vi "Main Loop.vi"(8 "error in (no error)":errorcluster, 10 "Chart Notifier":refnum<notifier>, 11 "Message Queues":T1) -> (0 "error out":errorcluster)   [LabVIEW 2018, in "Sonicator Module.lvlib" / "Sonicator Module Engine.lvlib"]
uses:
  Sonicator Module Engine.lvlib
  Sonicator Message Queues.ctl
  support/Message Queue/Message Cluster.ctl
  Feed Module/Controls/Sonicator Module Display.ctl
  Feed Module/Controls/Sonicator Module State Cluster.ctl
  Pump Module Folder/Measure Instrument/State Enum.ctl
  Feed Module/Controls/Sonicator Module Config Cluster.ctl
  <vilib>/Utility/miscctls.llb/LVPoint32TypeDef.ctl
  Feed Module/Controls/Sonicator Module Settings Cluster.ctl
  Sonic Systems P100/Sonic Systems P100 Settings.ctl
  <vilib>/Platform/TimedLoop/XDataNode/timing_clust.ctl
  <vilib>/Platform/TimedLoop/XDataNode/nitl_modes.ctl
  <vilib>/Platform/TimedLoop/XDataNode/wakeup.ctl
  Tag VIs/Tag FGV Operation Enum.ctl
  support/Message Queue/Enqueue Message (Single).vi
  <vilib>/Platform/TimedLoop/XDataNode/XDataNode.xnode
  support/Message Queue/Message Queue.lvlib
  <vilib>/Platform/TimedLoop/XDataNode/XDNodeRunTimeDep.lvlib
  Sonicator Module.lvlib
  Shared Variables/Dynamic Shared Variables.lvlib
  support/Support Library.lvlib
  Sonic Systems P100/Sonic Systems P100.lvlib
  Pump Module Folder/Measure Instrument/Pump Module Engine.lvlib
panel:
  out "Period (s) 2":dbl format="%_4g"
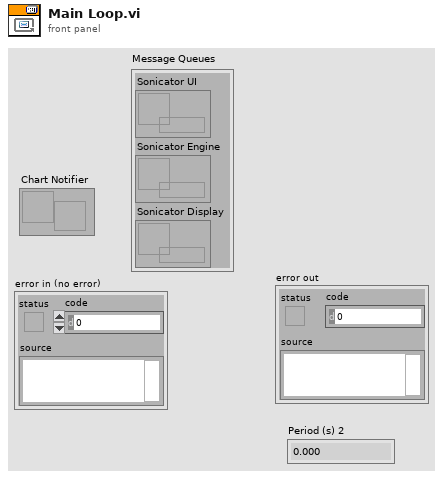
[diagram p1: front panel]
types:
  T1 = typedef "Sonicator Module.lvlib/Sonicator Message Queues.ctl" = cluster{"Sonicator UI":refnum<queue>, "Sonicator Engine":refnum<queue>, "Sonicator Display":refnum<queue>}
  T2 = typedef "XDNodeRunTimeDep.lvlib/timing_clust.ctl" = cluster{"Expected End [f-1]":u64, "Actual End [f-1]":u64, "Finished Late? [f-1]":bool, "Expected End [i-1]":u64, "Actual End [i-1]":u64, "Finished Late? [i-1]":bool, "Expected Start [i]":u64, "Actual Start [i]":u64, "Expected Start [f]":u64, "Actual Start [f]":u64, "Source Name":string, "Structure Name":string, "Period":i64, "Deadline":i64, "Offset":i64, "Start":i64, "Priority":i32, "Timeout":i32, "Mode":T3, "Wakeup Reason":T4, "Error":errorcluster, "Source Type":string, "Secondary Source Type":string, "Global End Time":u64, "Global Start Time":u64, "Frame Duration":u64, "Iteration Duration":u64, "Assigned CPU":i32, "I/O Scan Engine Mode":u32}
  T3 = typedef "XDNodeRunTimeDep.lvlib/nitl_modes.ctl" = enum32{"No Change", "Process missed periods, maintain original phase", "Discard missed periods, maintain original phase", "Process missed periods, ignore original phase", "Discard missed periods, ignore original phase"}
  T4 = typedef "XDNodeRunTimeDep.lvlib/wakeup.ctl" = enum32{"Normal", "Aborted", "Asynchronous wakeup", "Timing source error", "Timed loop error", "Timeout"}
  T5 = cluster{"enable? (F)":bool, "name":string, "alarm on":bool, "priority":u32, "ack type":enum16{"Auto", "User", "None", "Each Occurrence"}, "area":string, "description":string, "log? (T)":bool}
  T6 = typedef "Tag FGV Operation Enum.ctl" = enum16{"Init", "Set Notification Queue", "Create Tag", "Commit", "Write Tag (Numeric)", "Write Tag (Boolean)", "Read All Tags", "Read One Tag", "Delete Tag Category", "Set Alarm Parameters (Numeric)", "Set Alarm Parameters (Boolean)", "Enable All Alarms", "Disable All Alarms", "Delete All Tags", "Read Alarms", "Ack Alarm", "Read Alarm Parameters (Numeric)", "Read Alarm Parameters (Boolean)"}
  T7 = enum32{"u32BitField", "bool", "double", "string", "int8", "uint8", "int16", "uint16", "int32", "uint32", "int64", "uint64", "single", "double waveform", "int16 waveform", "array of boolean", "array of int8", "array of uint8", "array of int16", "array of uint16", "array of int32", "array of uint32", "array of int64", "array of uint64", "array of single", "array of double", "array of double waveform", "array of int16 waveform", "array of string", "variant", "timestamp", "fixed point", "custom"}
  T8 = typedef "Pump Module.lvlib/Pump Module Engine.lvlib/State Enum.ctl" = enum16{"Measuring", "Idle", "Paused"}
  T9 = enum16{"Off", "On", "Not Initialized", "Over Cutoff"}
  T10 = typedef "Sonicator Module.lvlib/Sonicator Module Config Cluster.ctl" = cluster{"GUID":string, "Drop Coords":T11, "Process Name":string, "User name":string, "Queue Name":string, "Settings":T12, "Load Count":i32}
  T11 = typedef "LVPoint32TypeDef.ctl" = cluster{"Horizontal":i32, "Vertical":i32}
  T12 = typedef "Sonicator Module.lvlib/Sonicator Module Settings Cluster.ctl" = cluster{"Cycle Period":dbl, "Sonicator Type":string, "SS P100 Settings":T13, "Setpoint (µm)":dbl, "Cutoff (W)":dbl}
  T13 = typedef "Sonic Systems P100.lvlib/Sonic Systems P100 Settings.ctl" = cluster{"VISA resource name":refnum<visa-resource-name>, "Simulated?":bool}
  T14 = typedef "Sonicator Module.lvlib/Sonicator Module State Cluster.ctl" = cluster{"State":T8, "Start Time":timestamp, "Current Time":timestamp, "Sonicator Module Config":T10, "Output Error":bool, "Log Started":bool, "First Iteration":bool, "Data":cluster{"Sonicator Amp Value":dbl, "Sonicator Power Value":dbl}, "Sonicator On?":enum16{"Off", "On", "Not Initialized", "Over Cutoff"}}
  T15 = typedef "Sonicator Module.lvlib/Sonicator Module Display.ctl" = cluster{"Sonicator On?":enum16{"Off", "On", "Not Initialized", "Over Cutoff"}, "Sonicator Amp Value":dbl, "Sonicator Power Value":dbl, "Cycle Period":dbl}
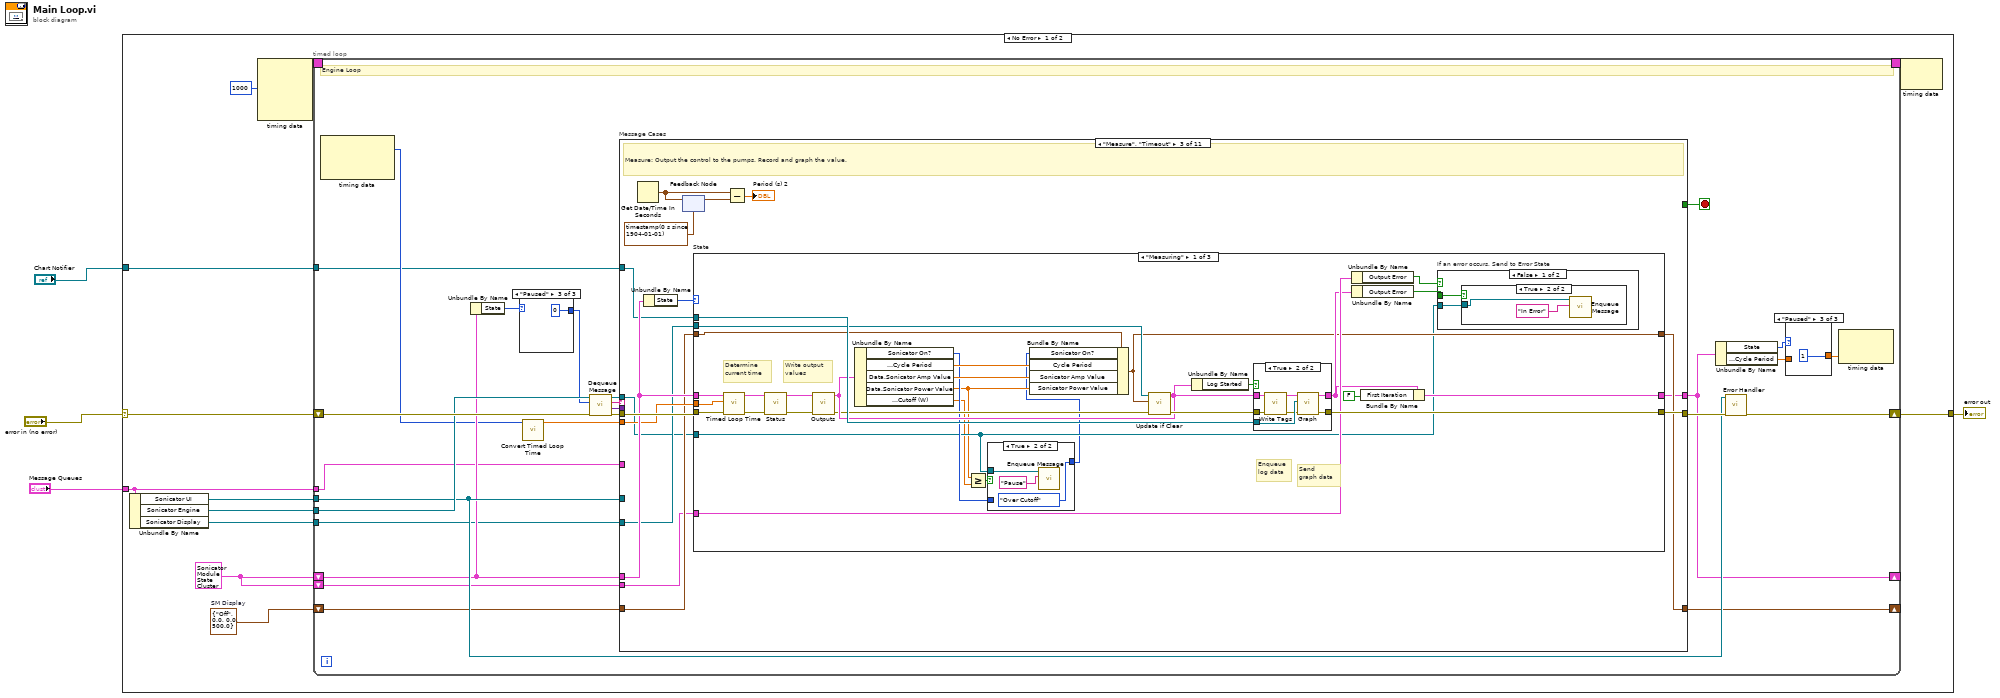
[diagram p0: block diagram]
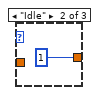
[diagram p3: hidden frame]
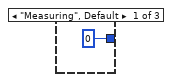
[diagram p4: hidden frame]
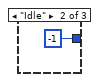
[diagram p5: hidden frame]
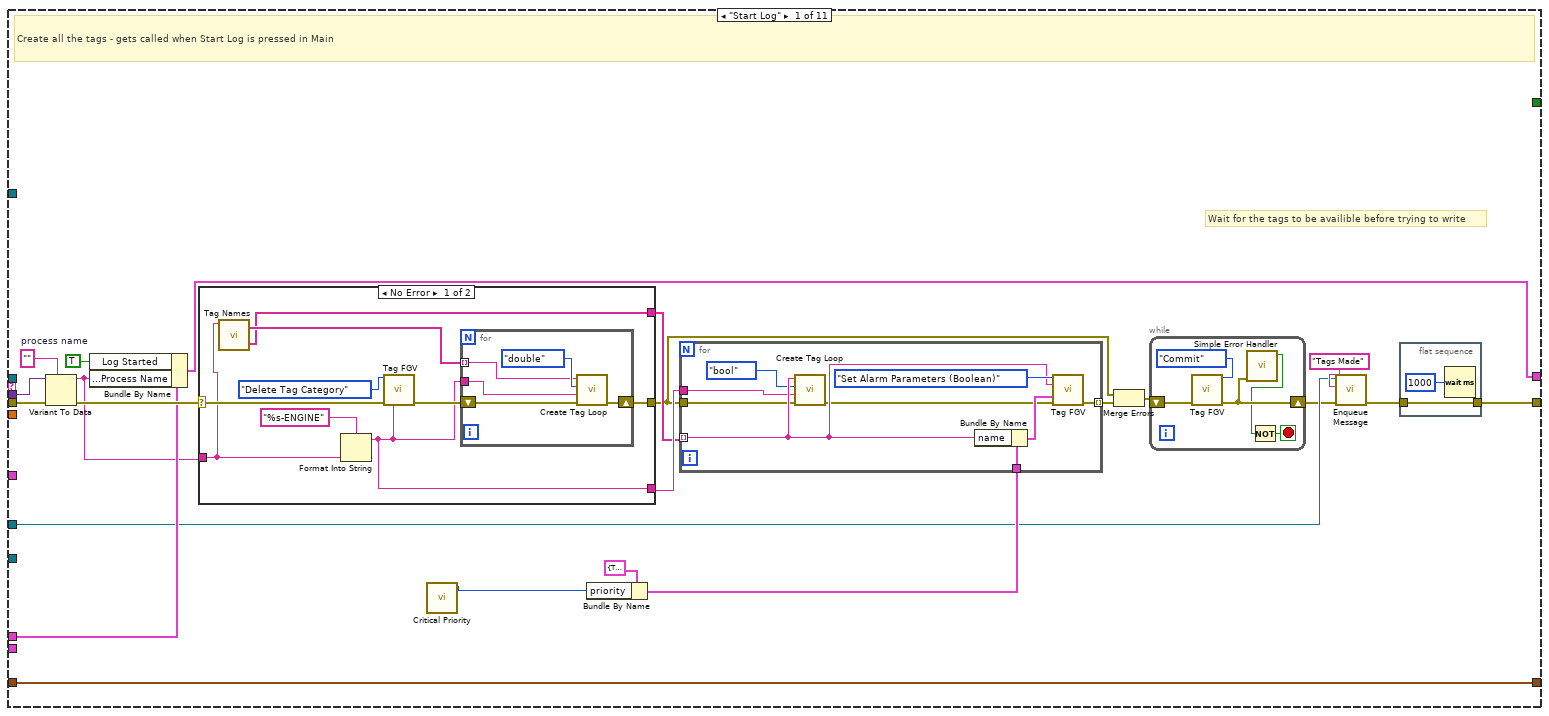
[diagram p6: hidden frame]
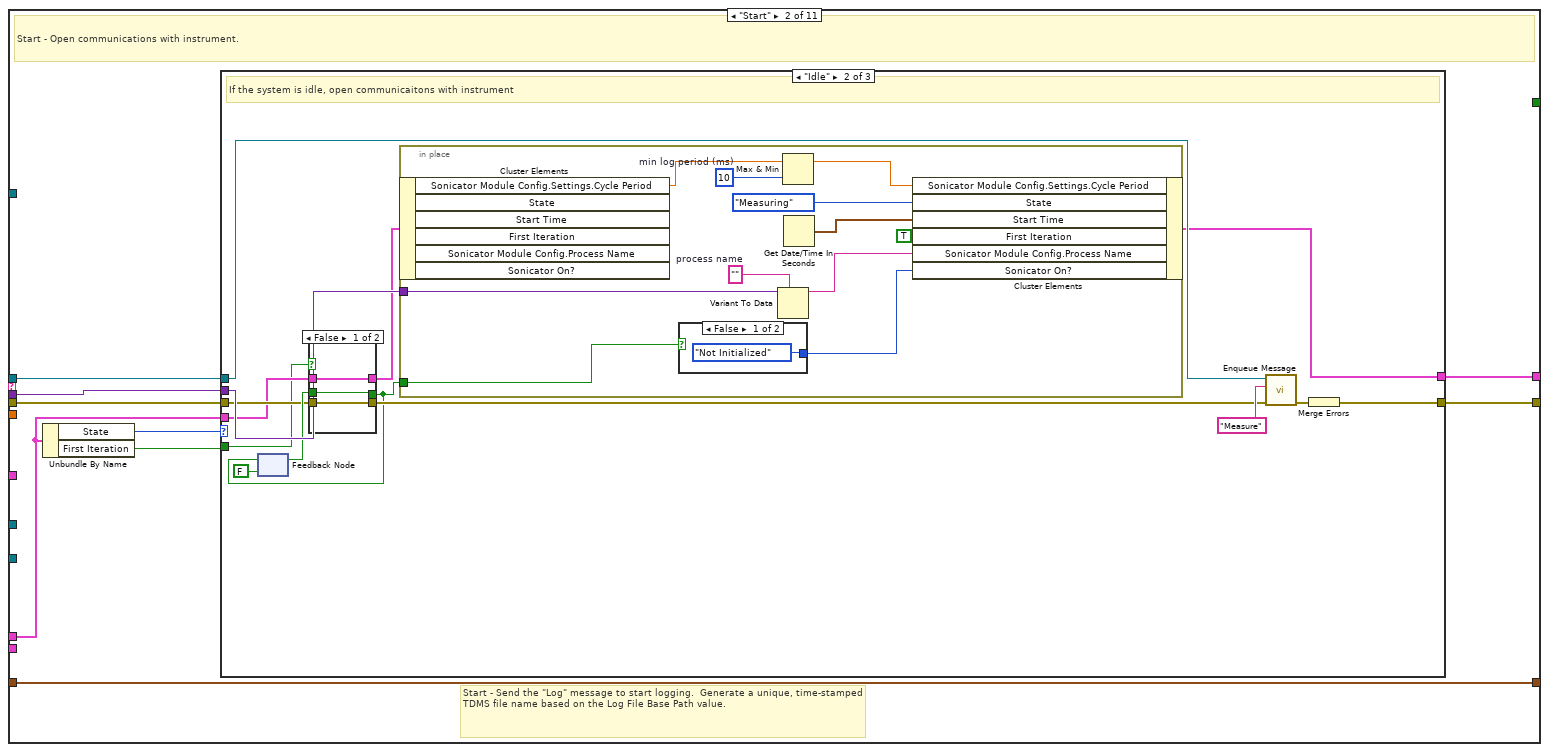
[diagram p8: hidden frame]
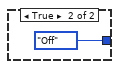
[diagram p10: hidden frame]
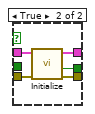
[diagram p11: hidden frame]
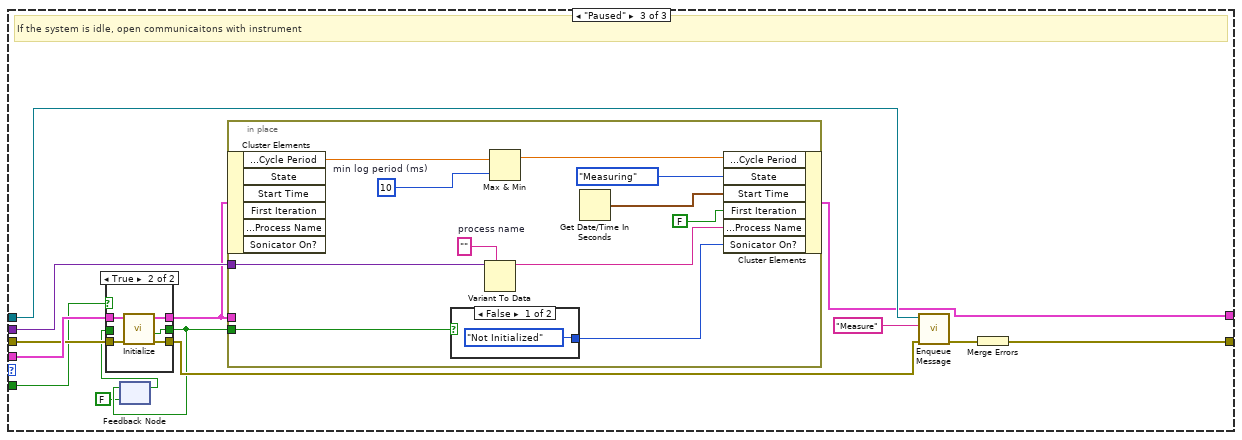
[diagram p12: hidden frame]
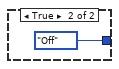
[diagram p13: hidden frame]
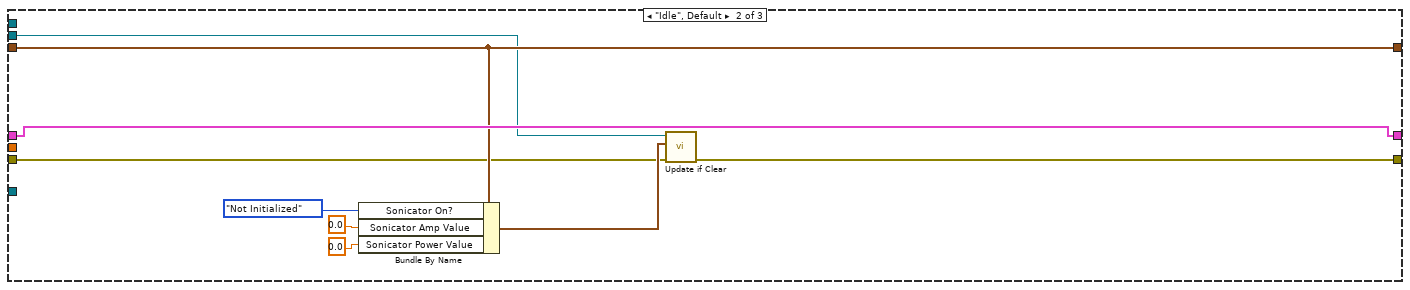
[diagram p19: hidden frame]
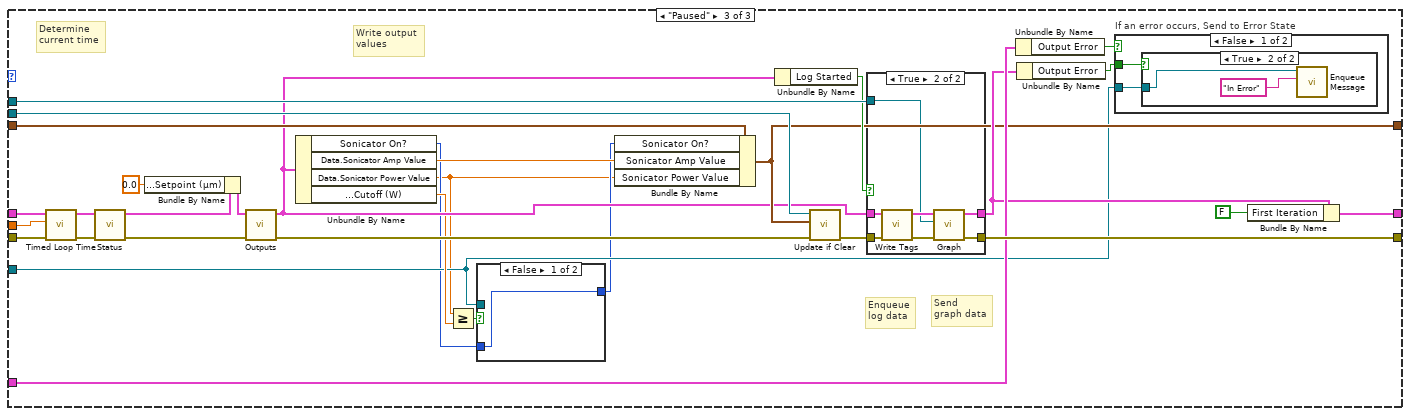
[diagram p20: hidden frame]
diagram:
  n1 = case shown="No Error" "error in (no error)" {
    selector: "error in (no error)" -> [w15 w423]
    tunnel: "Message Queues" -> [w11 _]
    tunnel: [w16 w423] -> w4
    tunnel: "Chart Notifier" -> [w9 _]
    frame No Error {
      w5 = T14 {"State"=enum."Idle", "Start Time"=timestamp(0 s since 1904-01-01), "Current Time"=timestamp(0 s since 1904-01-01), "Sonicator Module Config"={"GUID"="", "Drop Coords"={"Horizontal"=0, "Vertical"=0}, "Process Name"="", "User name"="", "Queue Name"="", "Settings"={"Cycle Period"=500.0, "Sonicator Type"="", "SS P100 Settings"={"VISA resource name"="", "Simulated?"=FALSE}, "Setpoint (µm)"=0.0, "Cutoff (W)"=0.0}, "Load Count"=0}, "Output Error"=FALSE, "Log Started"=FALSE, "First Iteration"=FALSE, "Data"={"Sonicator Amp Value"=0.0, "Sonicator Power Value"=0.0}, "Sonicator On?"=enum."Off"} ("Sonicator Module State Cluster")
      w6 = T15 {"Sonicator On?"=enum."Off", "Sonicator Amp Value"=0.0, "Sonicator Power Value"=0.0, "Cycle Period"=500.0}  # SM Display
      n2 = Unbundle By Name(w11) -> ("Sonicator UI"=w14:refnum<queue>, "Sonicator Engine"=w10:refnum<queue>, "Sonicator Display"=w8:refnum<queue>)
      n3 = node-c288(i64 1000 ("Period")) -> (w13:T2)  [unwired: 3 in]
      n4 = timed-loop {
        tunnel: w10 -> [w35]
        shift-right: [w17] -> _
        shift-left: w5 -> [w31]
        shift-right: [w33] -> w16
        shift-left: w15 -> [w40]
        tunnel: w14 -> [w32]
        timing: w13 -> [_]
        timing-out: [_] -> w12
        tunnel: w11 -> [w23]
        tunnel: w9 -> [w22]
        tunnel: w8 -> [w21]
        shift-right: [w20] -> _
        shift-left: w6 -> [w19]
        shift-left: w5 -> [w18]
        stop <- w41 stop-if-true
        # "Engine Loop"
        n5 = node-c288() -> (w25:i64)  [unwired: 1 in, 2 out]
        n6 = Unbundle By Name(w31) -> ("State"=w30:T8)
        n7 = case shown="\"Paused\"" w30 {
          tunnel: [0 ("timeout in ms (-1)") -1 ("timeout in ms (-1)") 0 ("timeout in ms (-1)")] -> w29
          frame "Measuring", Default {
          }
          frame "Idle" {
          }
          frame "Paused" {
          }
        }
        n8 = call "Convert Timed Loop Time.vi"("Actual Start [i]"=w25) -> ("ET since start (s)"=w24:dbl)  [unwired: 10 in]
        n9 = call "Dequeue Message.vi"("error in (no error)"=w40, "timeout in ms (-1)"=w29, "Message Queue"=w35) -> ("error out"=w39:errorcluster, "Message Data"=w37:variant, "Message"=w38:string, "dup Message Queue"=w36:refnum<queue>)  [unwired: 5 in]
        n10 = case "Message Cases" shown="\"Measure\", \"Timeout\"" w38 {
          selector: w38 -> [_ _ _ _ _ _ _ _ _ _ w412]
          tunnel: w36 -> [_ w113 w190 _ _ _ w366 _ w385 _ _]
          tunnel: w39 -> [w59 w112 w200 w312 w338 w360 w369 w376 w380 w410 _]
          tunnel: [w55 w114 w201 w307 w335 w357 w371 w375 w391 w409 w411] -> w34
          tunnel: w31 -> [w64 w109 w199 w314 w339 w358 w362 w373 w381 w407 w417]
          tunnel: [w53 w106 w188 w313 w328 w356 w362 w373 w392 w405 w417] -> w17
          tunnel: [_ _ _ _ _ _ TRUE _ _ _ _] -> w41
          tunnel: w37 -> [w73 w110 _ _ _ w361 _ _ _ _ _]
          tunnel: w32 -> [w61 _ _ w316 _ _ w370 _ _ _ _]
          tunnel: w24 -> [_ _ w198 _ _ _ _ _ _ _ _]
          tunnel: w23 -> [_ _ _ _ _ _ _ _ _ _ _]
          tunnel: w22 -> [_ _ w194 _ _ _ _ _ _ _ _]
          tunnel: w21 -> [_ _ w193 w310 w337 _ _ _ w384 _ _]
          tunnel: w19 -> [w74 w108 w192 w309 w336 w359 w363 w374 w390 w408 w418]
          tunnel: [w74 w108 w191 w309 w336 w359 w363 w374 w383 w408 w418] -> w20
          tunnel: w18 -> [_ _ w189 _ _ _ _ _ _ _ _]
          frame "Start Log" {
            w72 = ""  # process name
            # "Wait for the tags to be availible before trying to write"
            # "Create all the tags - gets called when Start Log is pressed in Main"
            n11 = Variant To Data(error in=w59, type=w72, Variant=w73) -> (data=w60:string, error out=w71:errorcluster)
            n12 = Bundle By Name(cluster=w64, "Log Started"=TRUE, "Sonicator Module Config.Process Name"=w60) -> (w53:T14)
            n13 = case shown="No Error" w71 {
              selector: w71 -> [w96 w105]
              tunnel: [w99 w105] -> w54
              tunnel: [w94 _] -> w67
              tunnel: [w92 _] -> w66
              tunnel: w60 -> [w91 _]
              frame No Error {
                n14 = call "Tag Names.vi"("Process Name"=w91) -> ("All Boolean Tags"=w92:string[], "All  Numeric Tags"=w93:string[])  [unwired: 8 in, 1 out]
                n15 = Format Into String(format string="%s-ENGINE", w91) -> (resulting string=w94:string)  [unwired: 2 in, 1 out]
                n16 = call "Tag FGV.vi"("Operation"=Tag_FGV_Operation_Enum."Delete Tag Category", "error in (no error)"=w96, "Tag Category"=w94) -> ("error out"=w95:errorcluster)  [unwired: 5 in, 7 out]
                n17 = for {
                  shift-right: [w100] -> w99
                  shift-left: w95 -> [w101]
                  tunnel: w94 -> [w102]
                  tunnel: w93 -> [w103] mode=indexing
                  n18 = call "Create Tag Loop.vi"("error in (no error)"=w101, "Tag Category"=w102, "data type"=T7."double", "Tag Name"=w103) -> ("error out"=w100:errorcluster)  [unwired: 7 in]
                }
              }
              frame Error {
              }
            }
            n19 = call "Critical Priority.vi"() -> ("critical priority"=w70:i32)  [unwired: 11 in]
            n20 = Bundle By Name(cluster=T5 {"enable? (F)"=TRUE, "name"="Boolean", "alarm on"=TRUE, "priority"=1, "ack type"=enum."Each Occurrence", "area"="a", "description"="", "log? (T)"=TRUE} ("Boolean alarm settings"), "priority"=w70) -> (w68:T5)
            n21 = for {
              tunnel: w68 -> [w90]
              tunnel: [w89] -> w65 mode=indexing
              tunnel: w66 -> [w86] mode=indexing
              tunnel: w54 -> [w83]
              tunnel: w67 -> [w84]
              n22 = call "Create Tag Loop.vi"("error in (no error)"=w83, "Tag Category"=w84, "data type"=T7."bool", "Tag Name"=w86) -> ("error out"=w82:errorcluster)  [unwired: 7 in]
              n23 = Bundle By Name(cluster=w90, "name"=w86) -> (w88:T5)
              n24 = call "Tag FGV.vi"("Operation"=Tag_FGV_Operation_Enum."Set Alarm Parameters (Boolean)", "Tag Name"=w86, "Data"=w88, "error in (no error)"=w82) -> ("error out"=w89:errorcluster)  [unwired: 4 in, 7 out]
            }
            n25 = Merge Errors(w54, w65) -> (w58:errorcluster)
            n26 = while {
              shift-right: [w79] -> w57
              shift-left: w58 -> [w80]
              stop <- w77 stop-if-true
              n27 = call "Tag FGV.vi"("Operation"=Tag_FGV_Operation_Enum."Commit", "error in (no error)"=w80) -> ("error out"=w79:errorcluster)  [unwired: 6 in, 7 out]
              n28 = call <vilib>:"Simple Error Handler.vi"("error in (no error)"=w79) -> ("error?"=w78:bool)  [unwired: 4 in, 4 out]
              n29 = Not(x=w78) -> (.not. x?=w77:bool)
            }
            n30 = call-poly "Enqueue Message.vi"("error in (no error)"=w57, "Message"="Tags Made", "Message Queue"=w61) -> ("error out"=w56:errorcluster)  [unwired: 7 in, 1 out]
            n31 = flat-sequence {
              tunnel: [w75] -> w55
              tunnel: w56 -> [w75]
              frame #0 {
                n32 = Wait (ms)(milliseconds to wait=u32 1000) -> ()  [unwired: 1 out]
              }
            }
          }
          frame "Start" {
            # "Start - Send the \"Log\" message to start logging.  Generate a unique, time-stamped TDMS file name based on the Log File Base Path value."
            # "Start - Open communications with instrument."
            n33 = Unbundle By Name(w109) -> ("State"=w111:T8, "First Iteration"=w107:bool)
            n34 = case shown="\"Paused\"" w111 {
              tunnel: [w115 w130 w165] -> w114
              tunnel: w113 -> [_ w127 w162]
              tunnel: w112 -> [w115 w124 w159]
              tunnel: w109 -> [w116 w123 w160]
              tunnel: [w116 w118 w153] -> w106
              tunnel: w110 -> [_ w126 w161]
              tunnel: w107 -> [_ w120 w155]
              frame "Measuring", Default {
                # "The system is already running. Ignore the \"Start\" message."
              }
              frame "Idle" {
                # "If the system is idle, open communicaitons with instrument"
                n35 = feedback #1(FALSE ("Initialized")) -> (w125:bool)
                n36 = case shown="False" w120 {
                  tunnel: w124 -> [w146 w147]
                  tunnel: w123 -> [w144 w148]
                  tunnel: [w144 w151] -> w119
                  tunnel: [w146 w150] -> w122
                  tunnel: [w145 w149] -> w121
                  tunnel: w125 -> [w145 _]
                  frame False {
                  }
                  frame True {
                    n37 = call "Initialize.vi"("error in (no error)"=w147, "Sonicator Module State Cluster"=w148) -> ("error out"=w150:errorcluster, "Initialized"=w149:bool, "Sonicator Module State Cluster"=w151:T14)  [unwired: 7 in]
                  }
                }
                n38 = feedback-in #1(w121) -> ()
                n39 = in-place {
                  in-place-border: w126 -> [w139]
                  in-place-border: w121 -> [w138]
                  w140 = ""  # process name
                  w141 = 10  # min log period (ms)
                  n40 = in-place-cluster #2(w119) -> ("Sonicator Module Config.Settings.Cycle Period"=w137:dbl)  [unwired: 5 out]
                  n41 = case shown="False" w138 {
                    tunnel: [enum16{"Off", "On", "Not Initialized"}."Not Initialized" ("Pump On?") enum16{"Off", "On", "Not Initialized"}."Off" ("Pump On?")] -> w131
                    frame False {
                    }
                    frame True {
                    }
                  }
                  n42 = Variant To Data(type=w140, Variant=w139) -> (data=w132:string)  [unwired: 1 in, 1 out]
                  n43 = Max & Min(x=w137, y=w141) -> (max(x,y)=w136:dbl)  [unwired: 1 out]
                  n44 = Get Date/Time In Seconds() -> (seconds since 1Jan1904=w134:timestamp)
                  n45 = in-place-cluster #2("Sonicator Module Config.Settings.Cycle Period"=w136, "State"=State_Enum."Measuring", "Start Time"=w134, "First Iteration"=TRUE, "Sonicator Module Config.Process Name"=w132, "Sonicator On?"=w131) -> (w118:T14)
                }
                n46 = call-poly "Enqueue Message.vi"("error in (no error)"=w122, "Message"="Measure", "Message Queue"=w127) -> ("error out"=w128:errorcluster)  [unwired: 7 in, 1 out]
                n47 = Merge Errors(w128) -> (w130:errorcluster)
              }
              frame "Paused" {
                # "If the system is idle, open communicaitons with instrument"
                n48 = feedback #3(FALSE ("Initialized")) -> (w156:bool)
                n49 = case shown="False" w155 {
                  tunnel: w159 -> [w180 w185]
                  tunnel: w160 -> [w181 w186]
                  tunnel: [w181 w182] -> w154
                  tunnel: [w180 w183] -> w158
                  tunnel: [w179 w184] -> w157
                  tunnel: w156 -> [w179 _]
                  frame False {
                  }
                  frame True {
                    n50 = call "Initialize.vi"("error in (no error)"=w185, "Sonicator Module State Cluster"=w186) -> ("error out"=w183:errorcluster, "Initialized"=w184:bool, "Sonicator Module State Cluster"=w182:T14)  [unwired: 7 in]
                  }
                }
                n51 = feedback-in #3(w157) -> ()
                n52 = in-place {
                  in-place-border: w161 -> [w174]
                  in-place-border: w154 -> [_]
                  in-place-border: w157 -> [w173]
                  w175 = ""  # process name
                  w176 = 10  # min log period (ms)
                  n53 = in-place-cluster #4(w154) -> ("Sonicator Module Config.Settings.Cycle Period"=w172:dbl)  [unwired: 5 out]
                  n54 = case shown="False" w173 {
                    tunnel: [enum16{"Off", "On", "Not Initialized"}."Not Initialized" ("Pump On?") enum16{"Off", "On", "Not Initialized"}."Off" ("Pump On?")] -> w166
                    frame False {
                    }
                    frame True {
                    }
                  }
                  n55 = Variant To Data(type=w175, Variant=w174) -> (data=w167:string)  [unwired: 1 in, 1 out]
                  n56 = Max & Min(x=w172, y=w176) -> (max(x,y)=w171:dbl)  [unwired: 1 out]
                  n57 = Get Date/Time In Seconds() -> (seconds since 1Jan1904=w169:timestamp)
                  n58 = in-place-cluster #4("Sonicator Module Config.Settings.Cycle Period"=w171, "State"=State_Enum."Measuring", "Start Time"=w169, "First Iteration"=FALSE, "Sonicator Module Config.Process Name"=w167, "Sonicator On?"=w166) -> (w153:T14)
                }
                n59 = call-poly "Enqueue Message.vi"("error in (no error)"=w158, "Message"="Measure", "Message Queue"=w162) -> ("error out"=w163:errorcluster)  [unwired: 7 in, 1 out]
                n60 = Merge Errors(w163) -> (w165:errorcluster)
              }
            }
          }
          frame "Measure", "Timeout" {
            # "Measure: Output the control to the pumps. Record and graph the value."
            n61 = Get Date/Time In Seconds() -> (seconds since 1Jan1904=w196:timestamp)
            n62 = Unbundle By Name(w199) -> ("State"=w202:T8)
            n63 = feedback-in #5(w196) -> ()
            n64 = feedback #5(timestamp(0 s since 1904-01-01) ("seconds since 1Jan1904")) -> (w197:timestamp)
            n65 = case "State" shown="\"Measuring\"" w202 {
              tunnel: w200 -> [w217 w251 w273]
              tunnel: w199 -> [w218 w258 w274]
              tunnel: [w232 w250 w286] -> w201
              tunnel: [w231 w258 w280] -> w188
              tunnel: w198 -> [w216 _ w275]
              tunnel: w194 -> [w229 _ w289]
              tunnel: w193 -> [w221 w253 w278]
              tunnel: w192 -> [w228 w257 w288]
              tunnel: [w220 w257 w277] -> w191
              tunnel: w190 -> [w206 _ w262]
              tunnel: w189 -> [w223 _ w284]
              frame "Measuring" {
                # "Determine\ncurrent time"
                # "Send\ngraph data"
                # "Enqueue\nlog data"
                # "Write output\nvalues"
                n66 = call "Timed Loop Time.vi"("error in (no error)"=w217, "ET since start (s)"=w216, "Sonicator Module State Cluster"=w218) -> ("error out"=w214:errorcluster, "Sonicator Module State Cluster"=w215:T14)  [unwired: 7 in]
                n67 = call "Status.vi"("error in (no error)"=w214, "Sonicator Module State Cluster"=w215) -> ("error out"=w212:errorcluster, "Sonicator Module State Cluster"=w213:T14)  [unwired: 8 in]
                n68 = call "Outputs.vi"("error in (no error)"=w212, "Sonicator Module State Cluster"=w213) -> ("error out"=w210:errorcluster, "Sonicator Module State Cluster"=w211:T14)  [unwired: 8 in]
                n69 = Unbundle By Name(w211) -> ("Sonicator On?"=w207:T9, "Sonicator Module Config.Settings.Cycle Period"=w227:dbl, "Data.Sonicator Amp Value"=w208:dbl, "Data.Sonicator Power Value"=w205:dbl, "Sonicator Module Config.Settings.Cutoff (W)"=w204:dbl)
                n70 = Greater Or Equal?(x=w205, y=w204) -> (x >= y?=w209:bool)
                n71 = case shown="True" w209 {
                  tunnel: w206 -> [_ w235]
                  tunnel: w207 -> [w233 _]
                  tunnel: [w233 T9."Over Cutoff" ("Sonicator On?")] -> w203
                  frame False {
                  }
                  frame True {
                    n72 = call-poly "Enqueue Message.vi"("Message"="Pause", "Message Queue"=w235) -> ()  [unwired: 8 in, 2 out]
                  }
                }
                n73 = Bundle By Name(cluster=w228, "Sonicator On?"=w203, "Cycle Period"=w227, "Sonicator Amp Value"=w208, "Sonicator Power Value"=w205) -> (w220:T15)
                n74 = call "Update if Clear.vi"("error in (no error)"=w210, "Message Data"=w220, "Queue in"=w221) -> ("error out"=w219:errorcluster)  [unwired: 8 in]
                n75 = Unbundle By Name(w211) -> ("Log Started"=w226:bool)
                n76 = case shown="True" w226 {
                  tunnel: [w241 w244] -> w232
                  tunnel: [w242 w243] -> w222
                  tunnel: w229 -> [_ w247]
                  tunnel: w211 -> [w242 w249]
                  tunnel: w219 -> [w241 w245]
                  frame False {
                  }
                  frame True {
                    n77 = call "Write Tags.vi"("error in (no error)"=w245, "Sonicator Module State Cluster"=w249) -> ("error out"=w246:errorcluster, "Sonicator Module State Cluster"=w248:T14)  [unwired: 8 in]
                    n78 = call "Graph.vi"("error in (no error)"=w246, "notifier out"=w247, "Sonicator Module State Cluster"=w248) -> ("error out"=w244:errorcluster, "Sonicator Module State Cluster"=w243:T14)  [unwired: 7 in]
                  }
                }
                n79 = Unbundle By Name(w223) -> ("Output Error"=w224:bool)
                n80 = Unbundle By Name(w222) -> ("Output Error"=w225:bool)
                n81 = Bundle By Name(cluster=w222, "First Iteration"=FALSE) -> (w231:T14)
                n82 = case "If an error occurs, Send to Error State" shown="False" w224 {
                  tunnel: w225 -> [w238 _]
                  tunnel: w206 -> [w237 _]
                  frame False {
                    n83 = case shown="True" w238 {
                      tunnel: w237 -> [_ w239]
                      frame False {
                      }
                      frame True {
                        n84 = call-poly "Enqueue Message.vi"("Message"="In Error", "Message Queue"=w239) -> ()  [unwired: 8 in, 2 out]
                      }
                    }
                  }
                  frame True {
                  }
                }
              }
              frame "Idle", Default {
                n85 = Bundle By Name(cluster=w257, "Sonicator On?"=enum16{"Off", "On", "Not Initialized"}."Not Initialized" ("Pump On?"), "Sonicator Amp Value"=0.0 ("Current Pump Speed"), "Sonicator Power Value"=0.0 ("Current Pump Pressure")) -> (w252:T15)
                n86 = call "Update if Clear.vi"("error in (no error)"=w251, "Message Data"=w252, "Queue in"=w253) -> ("error out"=w250:errorcluster)  [unwired: 8 in]
              }
              frame "Paused" {
                # "Determine\ncurrent time"
                # "Write output\nvalues"
                # "Send\ngraph data"
                # "Enqueue\nlog data"
                n87 = call "Timed Loop Time.vi"("error in (no error)"=w273, "ET since start (s)"=w275, "Sonicator Module State Cluster"=w274) -> ("error out"=w271:errorcluster, "Sonicator Module State Cluster"=w270:T14)  [unwired: 7 in]
                n88 = call "Status.vi"("error in (no error)"=w271, "Sonicator Module State Cluster"=w270) -> ("error out"=w268:errorcluster, "Sonicator Module State Cluster"=w272:T14)  [unwired: 8 in]
                n89 = Bundle By Name(cluster=w272, "Sonicator Module Config.Settings.Setpoint (µm)"=0.0 ("Configuration.Manual Entry")) -> (w269:T14)
                n90 = call "Outputs.vi"("error in (no error)"=w268, "Sonicator Module State Cluster"=w269) -> ("error out"=w267:errorcluster, "Sonicator Module State Cluster"=w266:T14)  [unwired: 8 in]
                n91 = Unbundle By Name(w266) -> ("Sonicator On?"=w261:T9, "Data.Sonicator Amp Value"=w265:dbl, "Data.Sonicator Power Value"=w259:dbl, "Sonicator Module Config.Settings.Cutoff (W)"=w264:dbl)
                n92 = Greater Or Equal?(x=w259, y=w264) -> (x >= y?=w263:bool)
                n93 = case shown="False" w263 {
                  tunnel: w262 -> [_ w292]
                  tunnel: w261 -> [w290 _]
                  tunnel: [w290 T9."Over Cutoff" ("Sonicator On?")] -> w260
                  frame False {
                  }
                  frame True {
                    n94 = call-poly "Enqueue Message.vi"("Message"="Pause", "Message Queue"=w292) -> ()  [unwired: 8 in, 2 out]
                  }
                }
                n95 = Bundle By Name(cluster=w288, "Sonicator On?"=w260, "Sonicator Amp Value"=w265, "Sonicator Power Value"=w259) -> (w277:T15)
                n96 = Unbundle By Name(w266) -> ("Log Started"=w279:bool)
                n97 = call "Update if Clear.vi"("error in (no error)"=w267, "Message Data"=w277, "Queue in"=w278) -> ("error out"=w276:errorcluster)  [unwired: 8 in]
                n98 = case shown="True" w279 {
                  tunnel: w289 -> [_ w299]
                  tunnel: w276 -> [w295 w302]
                  tunnel: [w295 w297] -> w286
                  tunnel: [w294 w296] -> w281
                  tunnel: w266 -> [w294 w301]
                  frame False {
                  }
                  frame True {
                    n99 = call "Write Tags.vi"("error in (no error)"=w302, "Sonicator Module State Cluster"=w301) -> ("error out"=w298:errorcluster, "Sonicator Module State Cluster"=w300:T14)  [unwired: 8 in]
                    n100 = call "Graph.vi"("error in (no error)"=w298, "notifier out"=w299, "Sonicator Module State Cluster"=w300) -> ("error out"=w297:errorcluster, "Sonicator Module State Cluster"=w296:T14)  [unwired: 7 in]
                  }
                }
                n101 = Unbundle By Name(w284) -> ("Output Error"=w283:bool)
                n102 = Unbundle By Name(w281) -> ("Output Error"=w285:bool)
                n103 = case "If an error occurs, Send to Error State" shown="False" w283 {
                  tunnel: w285 -> [w304 _]
                  tunnel: w262 -> [w303 _]
                  frame False {
                    n104 = case shown="True" w304 {
                      tunnel: w303 -> [_ w306]
                      frame False {
                      }
                      frame True {
                        n105 = call-poly "Enqueue Message.vi"("Message"="In Error", "Message Queue"=w306) -> ()  [unwired: 8 in, 2 out]
                      }
                    }
                  }
                  frame True {
                  }
                }
                n106 = Bundle By Name(cluster=w281, "First Iteration"=FALSE) -> (w280:T14)
              }
            }
            n107 = Subtract(x=w196, y=w197) -> (x-y=→"Period (s) 2":dbl)
          }
          frame "Stop" {
            # "Stop - Flush the message queue of any pending \"Log\" messages. Call 'Flush Data to Log File.vi' so any pending data is not lost."
            n108 = call <vilib>:"Clear Errors.vi"("error in (no error)"=w312) -> ("error out"=w311:errorcluster)  [unwired: 5 in, 1 out]
            n109 = Unbundle By Name(w314) -> ("State"=w315:T8)
            n110 = case shown="\"Measuring\", Default" w315 {
              tunnel: [w321 w327] -> w308
              tunnel: w311 -> [w319 w327]
              tunnel: w316 -> [w325 _]
              tunnel: w314 -> [w320 w326]
              tunnel: [w323 w326] -> w313
              frame "Measuring", Default {
                # "If the system is logging, stop logging."
                n111 = call "Close.vi"("error in (no error)"=w319, "Sonicator Module State Cluster"=w320) -> ("error out"=w317:errorcluster, "Sonicator Module State Cluster"=w318:T14)  [unwired: 8 in]
                n112 = Bundle By Name(cluster=w318, "State"=State_Enum."Idle") -> (w323:T14)
                n113 = call-poly "Enqueue Message.vi"("error in (no error)"=w317, "Message"="Logging Stopped", "Message Queue"=w325) -> ("error out"=w321:errorcluster)  [unwired: 7 in, 1 out]
              }
              frame "Idle" {
                # "The system is already idle. Ignore the \"Stop\" message."
              }
            }
            n114 = call "Update if Clear.vi"("error in (no error)"=w308, "Message Data"=w309, "Queue in"=w310) -> ("error out"=w307:errorcluster)  [unwired: 8 in]
          }
          frame "Pause" {
            # "Stop - Flush the message queue of any pending \"Log\" messages. Call 'Flush Data to Log File.vi' so any pending data is not lost."
            n115 = Unbundle By Name(w339) -> ("First Iteration"=w340:bool)  [unwired: 1 out]
            n116 = case shown="False" w340 {
              tunnel: w339 -> [w341 w347]
              tunnel: [w341 w349] -> w332
              tunnel: w338 -> [w342 w343]
              tunnel: [w342 w344] -> w333
              frame False {
              }
              frame True {
                # "If we start on a pause condition, initialize the pump"
                n117 = call "Initialize.vi"("error in (no error)"=w343, "Sonicator Module State Cluster"=w347) -> ("error out"=w344:errorcluster, "Initialized"=w346:bool, "Sonicator Module State Cluster"=w345:T14)  [unwired: 7 in]
                n118 = case shown="True" w346 {
                  tunnel: [enum16{"Off", "On", "Not Initialized"}."Not Initialized" ("Pump On?") enum16{"Off", "On", "Not Initialized"}."Off" ("Pump On?")] -> w350
                  tunnel: [_ FALSE] -> w348
                  frame False {
                  }
                  frame True {
                  }
                }
                n119 = Bundle By Name(cluster=w345, "Sonicator On?"=w350, "First Iteration"=w348) -> (w349:T14)
              }
            }
            n120 = call <vilib>:"Clear Errors.vi"("error in (no error)"=w333) -> ("error out"=w331:errorcluster)  [unwired: 5 in, 1 out]
            n121 = call "Pause.vi"("error in (no error)"=w331, "Sonicator Module State Cluster"=w332) -> ("error out"=w329:errorcluster, "Sonicator Module State Cluster"=w330:T14)  [unwired: 8 in]
            n122 = Bundle By Name(cluster=w330, "State"=State_Enum."Paused") -> (w328:T14)
            n123 = call "Update if Clear.vi"("error in (no error)"=w329, "Message Data"=w336, "Queue in"=w337) -> ("error out"=w335:errorcluster)  [unwired: 8 in]
          }
          frame "Update Settings" {
            # "New settings are available, update the current ones stored in the shift register with the settings sent as part of the message"
            n124 = Variant To Data(error in=w360, type=T10 {"GUID"="", "Drop Coords"={"Horizontal"=0, "Vertical"=0}, "Process Name"="", "User name"="", "Queue Name"="", "Settings"={"Cycle Period"=500.0, "Sonicator Type"="", "SS P100 Settings"={"VISA resource name"="", "Simulated?"=FALSE}, "Setpoint (µm)"=0.0, "Cutoff (W)"=0.0}, "Load Count"=0} ("Sonicator Module Config"), Variant=w361) -> (data=w355:T10, error out=w357:errorcluster)
            n125 = Bundle By Name(cluster=w358, "Sonicator Module Config"=w355) -> (w356:T14)
          }
          frame "Exit" {
            # "Release the Logging queue reference"
            # "Don't check the error out. The UI message queue may have already been released."
            # "Stop the VI"
            # "Exit - Send the Exit message to the UI Message Handler.  Call 'Flush Data to Log File.vi' so any pending data is not lost."
            n126 = Release Queue(queue=w366, error in (no error)=w369) -> (error out=w365:errorcluster)  [unwired: 1 in, 2 out]
            n127 = call-poly "Enqueue Message.vi"("Priority Message? (F)"=TRUE, "Message"="Exit", "Message Queue"=w370) -> ("error out"=w364:errorcluster)  [unwired: 7 in, 1 out]
            n128 = call <vilib>:"Clear Errors.vi"("error in (no error)"=w364) -> ()  [unwired: 5 in, 2 out]
            n129 = Merge Errors(w365) -> (w371:errorcluster)
          }
          frame "---Copy This Frame---" {
            # "Duplicate this frame when creating new messages.  Change this comment in the duplicated frame to describe this message."
            n130 = Merge Errors(w376) -> (w375:errorcluster)
          }
          frame "In Error" {
            # "If we have a disconnect Error we will go to this state, and attempt to reconnect and get back to the pre-error state"
            n131 = Merge Errors(w380) -> ()  [unwired: 1 out]
            n132 = call "Initialize.vi"("error in (no error)"=w380, "Sonicator Module State Cluster"=w381) -> ("error out"=w378:errorcluster, "Initialized"=w377:bool, "Sonicator Module State Cluster"=w379:T14)  [unwired: 7 in]
            n133 = Unbundle By Name(w379) -> ("Sonicator On?"=w386:T9, "Sonicator Module Config.Settings.Cycle Period"=w387:dbl, "Data.Sonicator Amp Value"=w388:dbl, "Data.Sonicator Power Value"=w389:dbl)
            n134 = Bundle By Name(cluster=w390, "Sonicator On?"=w386, "Cycle Period"=w387, "Sonicator Amp Value"=w388, "Sonicator Power Value"=w389) -> (w383:T15)
            n135 = call "Update if Clear.vi"("error in (no error)"=w378, "Message Data"=w383, "Queue in"=w384) -> ("error out"=w382:errorcluster)  [unwired: 8 in]
            n136 = case shown="False" w377 {
              tunnel: w385 -> [w397 w401]
              tunnel: w382 -> [w396 w400]
              tunnel: [w394 w403] -> w392
              tunnel: w379 -> [w394 w403]
              tunnel: [w393 w399] -> w391
              frame False {
                n137 = Wait (ms)(milliseconds to wait=u32 5000) -> ()  [unwired: 1 out]
                n138 = call-poly "Enqueue Message.vi"("error in (no error)"=w396, "Message"="In Error", "Message Queue"=w397) -> ("error out"=w393:errorcluster)  [unwired: 7 in, 1 out]
              }
              frame True {
                n139 = call-poly "Enqueue Message.vi"("error in (no error)"=w400, "Message"="Measure", "Message Queue"=w401) -> ("error out"=w399:errorcluster)  [unwired: 7 in, 1 out]
              }
            }
          }
          frame "Initialize" {
            # "Duplicate this frame when creating new messages.  Change this comment in the duplicated frame to describe this message."
            n140 = Merge Errors(w410) -> (w409:errorcluster)
            n141 = Bundle By Name(cluster=w407, "Log Started"=FALSE, "First Iteration"=TRUE) -> (w405:T14)
          }
          frame Default {
            # "'Default' case only runs if there is a message that isn't defined in any of the other cases.  Output a programming error."
            n142 = Concatenate Strings("The invalid message string " ("string"), w412, " was received in the Pump Module Engine." ("string")) -> (w413:string)
            n143 = Bundle By Name(cluster=errorcluster {"status"=TRUE, "code"=1, "source"=""} ("error constant"), "source"=w413) -> (w411:errorcluster)
          }
        }
        n144 = Unbundle By Name(w17) -> ("State"=w28:T8, "Sonicator Module Config.Settings.Cycle Period"=w26:dbl)
        n145 = call "Error Handler.vi"("error in (no error)"=w34, "Message Queue"=w32) -> ("dup error in"=w33:errorcluster)  [unwired: 8 in, 1 out]
        n146 = case shown="\"Paused\"" w28 {
          tunnel: [w42 1 1] -> w27
          tunnel: w26 -> [w42 _ _]
          frame "Measuring" {
          }
          frame "Idle" {
          }
          frame "Paused" {
          }
        }
        n147 = node-c288(w27) -> ()  [unwired: 1 in, 1 out]
      }
      n148 = node-c288(w12) -> ()  [unwired: 1 out]
    }
    frame Error {
    }
  }
  "error out" <- w4
